vi "MotorControl_TestStand.vi"(6 "error in (no error)":errorcluster, 11 "Array":dbl[](array[numeric])) -> (3 "error out":errorcluster)   [LabVIEW 2019]
panel:
  out "error out 2":errorcluster
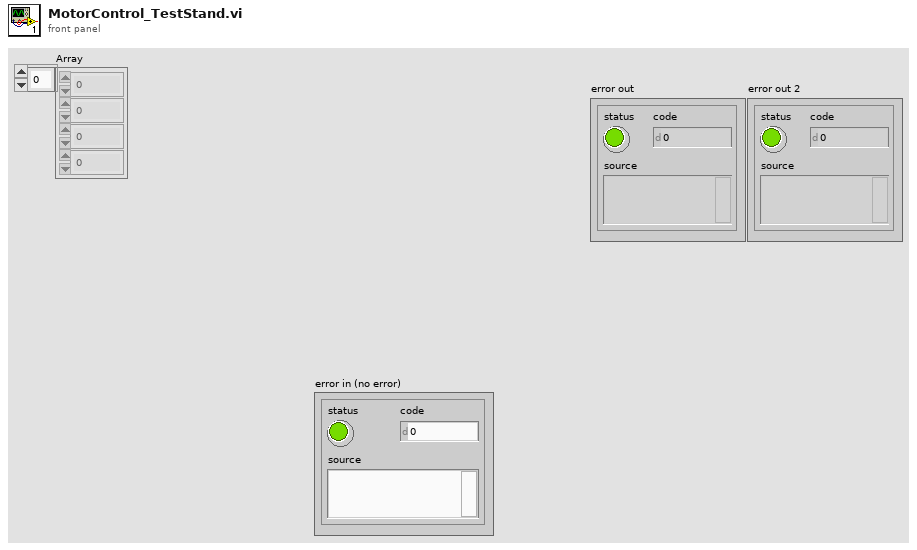
[diagram p1: front panel]
types:
  T1 = cluster{"Array[0]":dbl, "Array[1]":dbl, "Array[2]":dbl, "Array[3]":dbl, "Array[4]":dbl, "Array[5]":dbl, "Array[6]":dbl, "Array[7]":dbl, "Array[8]":dbl}
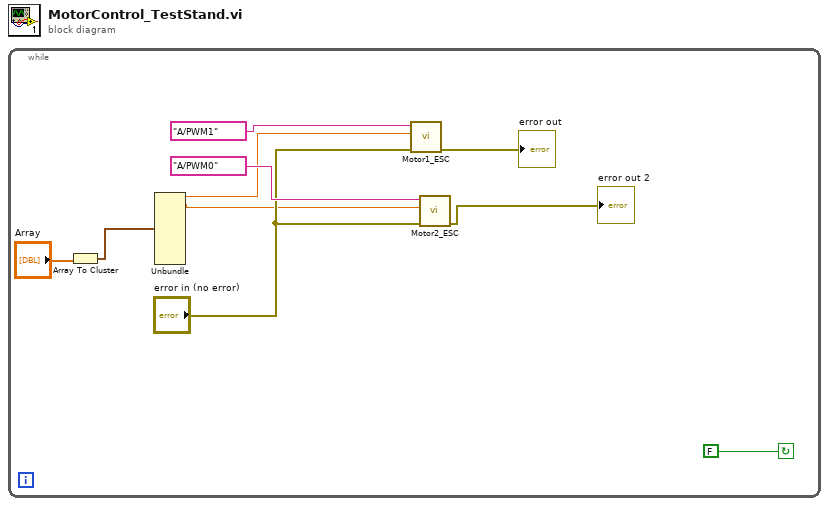
[diagram p0: block diagram]
diagram:
  n1 = while {
    stop <- FALSE continue-if-true
    n2 = Array To Cluster(array="Array") -> (cluster=w3:T1)
    n3 = Unbundle(w3) -> ("Array[0]"=w2:dbl, "Array[1]"=w1:dbl)  [unwired: 7 out]
    n4 = call "Motor1_ESC.vi"("error in (no error)"="error in (no error)", "Percent Power"=w2, "Channel Name"=tag "A/PWM1") -> ("error out"=→"error out":errorcluster)  [unwired: 8 in]
    n5 = call "Motor2_ESC.vi"("error in (no error)"="error in (no error)", "Percent Power"=w1, "Channel Name"=tag "A/PWM0") -> ("error out"=→"error out 2":errorcluster)  [unwired: 8 in]
  }
